vi "Read LibraryDirectories.vi"(11 "ProjectItem in":refnum<class "ProjectItem.lvclass">) -> (2 "LibraryDirectories":T1, 3 "ProjectItem out":refnum<class "ProjectItem.lvclass">)   [LabVIEW 2016, in "ProjectItem.lvclass"]
uses:
  ProjectItem.lvclass
  Typedefs/LibraryDirectories.ctl
  ProjectItem.lvclass/ProjectItem.ctl
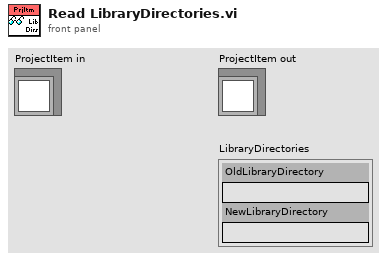
[diagram p1: front panel]
types:
  T1 = typedef "LibraryDirectories.ctl" = cluster{"OldLibraryDirectory":string, "NewLibraryDirectory":string}
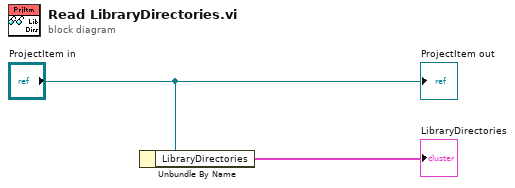
[diagram p0: block diagram]
diagram:
  n1 = Unbundle By Name("ProjectItem in") -> ("LibraryDirectories"=→"LibraryDirectories":T1)
  "ProjectItem out" <- "ProjectItem in"
